vi "Shot Complete--Const.vi"() -> (3 "Shot Complete Message":string)   [LabVIEW 2017, in "Communications Library.lvlib"]
uses:
  Communications Library.lvlib
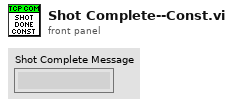
[diagram p1: front panel]
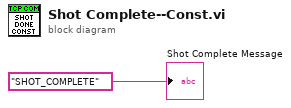
[diagram p0: block diagram]
diagram:
  "Shot Complete Message" <- "SHOT_COMPLETE" ("data in")
